vi "crio_RT_HX711.vi"() -> ()   [LabVIEW 2019]
uses:
  <vilib>/FPGAPlugInAG/cRIO-9074/niLvFpga_Open_cRIO-9074.vi
  <vilib>/rvi/interface/common/dynamic/niFpgaDynamicAddResources.vi
  <vilib>/Utility/error.llb/Error Cluster From Error Code.vi
  <vilib>/rvi/errors/niLvFpgaAdjustHostInterfaceError.vi
  <vilib>/FPGAPlugInAG/Dynamic/niLvFpga_Close_Dynamic.vi
  <vilib>/rvi/interface/nirviOpenFPGA/nirviOpenFPGA.xnode
  FPGA Bitfiles/gpass2_FPGATarget2_qweer_silS8sheR8k.lvbitx
  hx711/HX711.vi
  <vilib>/rvi/interface/nirviReadWriteControl/nirviReadWriteControl.xnode
  <vilib>/rvi/interface/nirviCloseFPGA/nirviCloseFPGA.xnode
  <vilib>/rvi/interface/Simulation/niFpgaSimulationCallBeginRW.vi
  NiFpgaLv.dll
  <vilib>/ptbypt/NI_PtbyPt.lvlib
panel:
  out "Offsetted Data":dbl(graph)
  out "Offsetted Data":dbl
  in  "Offset Bias":bool
  out "Computed Bias":dbl(graph)
  in  "Number of Samples for Offset Computation":i32=100
  out "Computed Bias":dbl format="%0.2f"
  out "Raw Data":i32(graph)
  in  "Gain/ChannelSelect":T1(ring)=enum."Channel A/Gain 64"
  out "HX711 Raw Data":i32
  in  "stop":bool
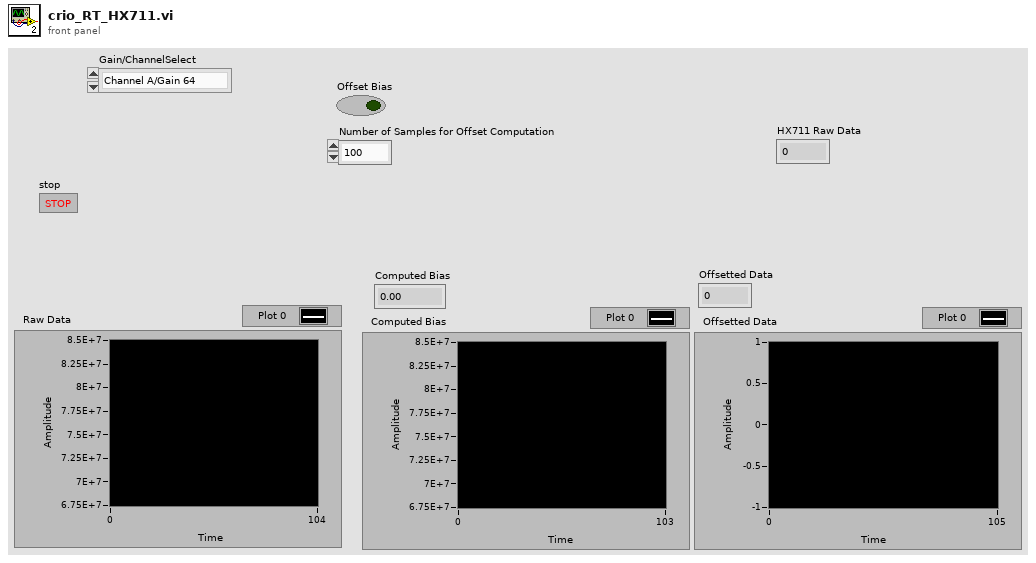
[diagram p1: front panel]
types:
  T1 = enum16{"Channel A/Gain 128", "Channel A/Gain 64", "Channel B/Gain 32"}
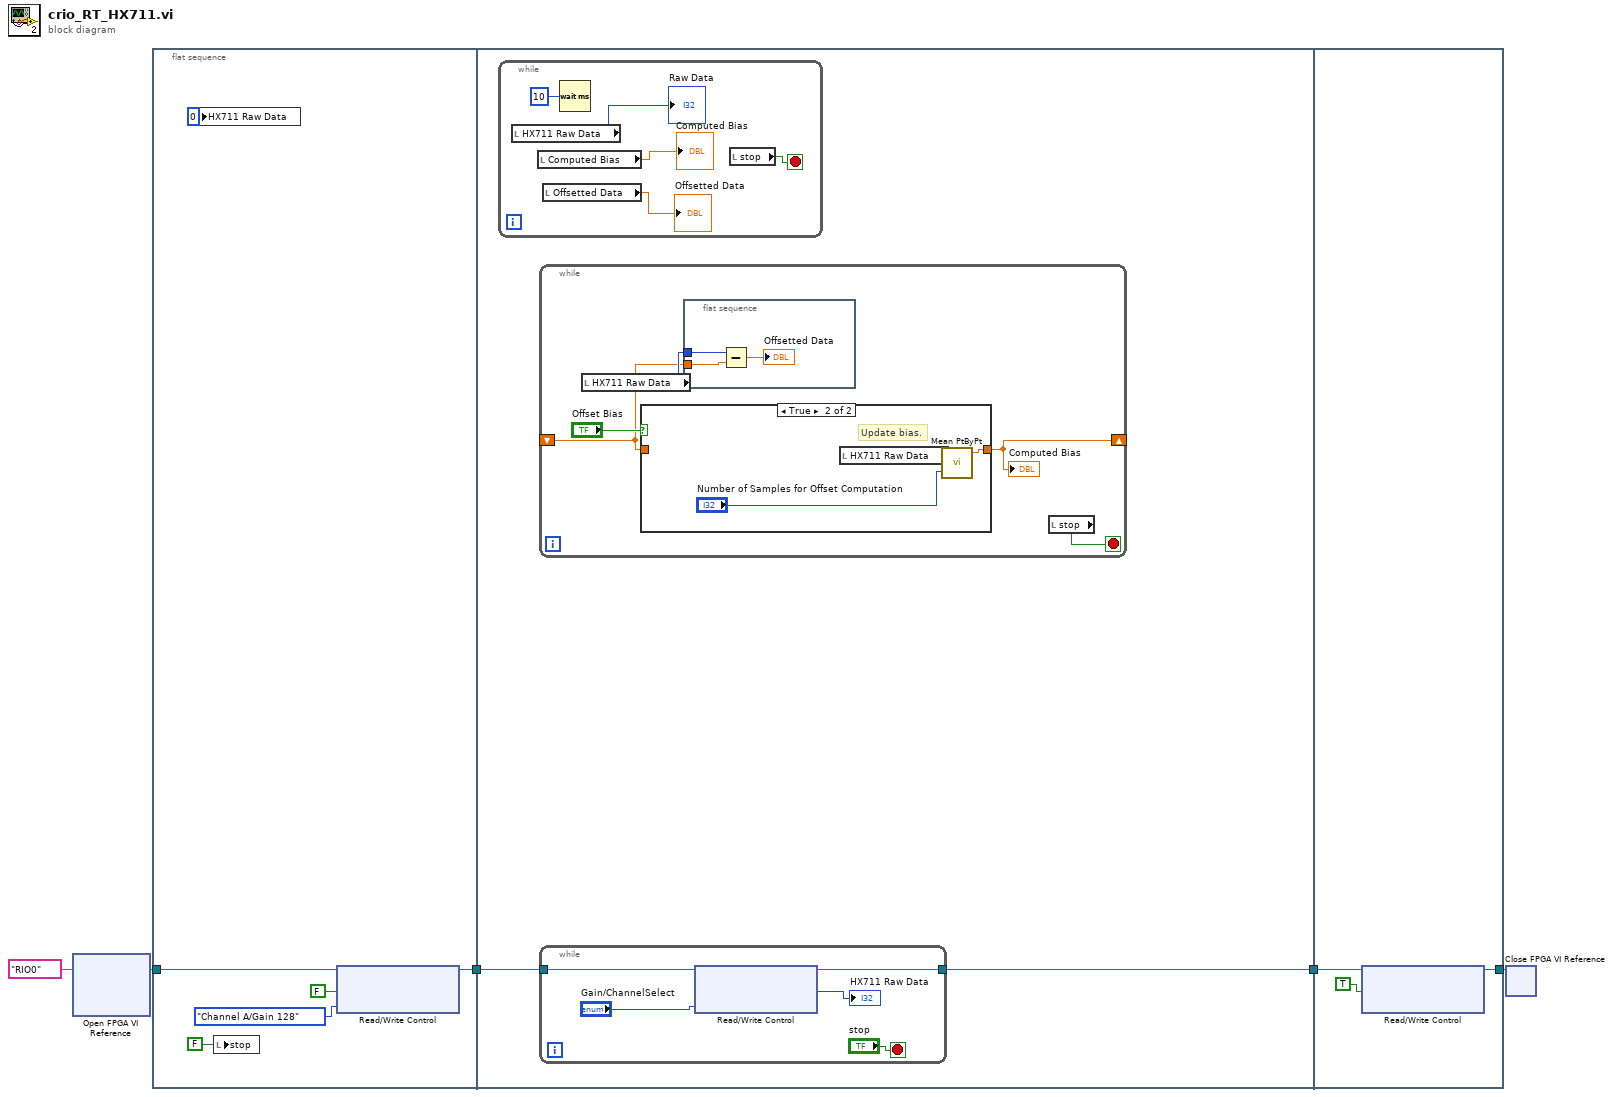
[diagram p0: block diagram]
diagram:
  n1 = xnode "Open FPGA VI Reference"("resource name"=tag "RIO0") -> ("FPGA VI Reference Out"=w4:refnum<k20>)  [unwired: 1 in, 1 out]
  n2 = flat-sequence {
    tunnel: w4 -> [w11]
    tunnel: [w9] -> w3
    tunnel: w3 -> [w12]
    tunnel: [w13] -> w2
    tunnel: w2 -> [w37]
    tunnel: [w36] -> w1
    frame #0 {
      n3 = local write "HX711 Raw Data"(0 ("Data")) -> ()
      n4 = local write "stop"(FALSE ("stop")) -> ()
      n5 = xnode "Read/Write Control"("FPGA VI Reference In"=w11, "stop"=FALSE, "Gain/ChannelSelect"=T1."Channel A/Gain 128") -> ("FPGA VI Reference Out"=w9:refnum<k20>)  [unwired: 1 in, 1 out]
    }
    frame #1 {
      n6 = while {
        stop <- w30 stop-if-true
        n7 = local read "HX711 Raw Data"() -> (→"Raw Data":i32)
        n8 = local read "Computed Bias"() -> (→"Computed Bias":dbl)
        n9 = local read "Offsetted Data"() -> (→"Offsetted Data":dbl)
        n10 = Wait (ms)(milliseconds to wait=u32 10) -> ()  [unwired: 1 out]
        n11 = local read "stop"() -> (w30:bool)
      }
      n12 = while {
        shift-right: [w16] -> _
        shift-left: _ -> [w14]
        stop <- w18 stop-if-true
        n13 = local read "HX711 Raw Data"() -> (w15:i32)
        n14 = case shown="True" "Offset Bias" {
          tunnel: [w22 w24] -> w16
          tunnel: w14 -> [w22 _]
          frame False {
            # "Stick with latest bias."
          }
          frame True {
            # "Update bias."
            n15 = local read "HX711 Raw Data"() -> (w25:i32)
            n16 = call <vilib>:"Mean PtByPt.vi"("x"=w25, "sample length"="Number of Samples for Offset Computation") -> ("mean"=w24:dbl)  [unwired: 2 in, 1 out]
          }
        }
        "Computed Bias" <- w16
        n17 = flat-sequence {
          tunnel: w15 -> [w21]
          tunnel: w14 -> [w20]
          frame #0 {
            n18 = Subtract(x=w21, y=w20) -> (x-y=→"Offsetted Data":dbl)
          }
        }
        n19 = local read "stop"() -> (w18:bool)
      }
      n20 = while {
        tunnel: w12 -> [w35]
        tunnel: [w32] -> w13
        stop <- "stop" stop-if-true
        n21 = xnode "Read/Write Control"("FPGA VI Reference In"=w35, "Gain/ChannelSelect"="Gain/ChannelSelect") -> ("FPGA VI Reference Out"=w32:refnum<k20>, "Data"=→"HX711 Raw Data":i32)  [unwired: 1 in, 1 out]
      }
    }
    frame #2 {
      n22 = xnode "Read/Write Control"("FPGA VI Reference In"=w37, "stop"=TRUE) -> ("FPGA VI Reference Out"=w36:refnum<k20>)  [unwired: 2 in, 1 out]
    }
  }
  n23 = xnode "Close FPGA VI Reference"("FPGA VI Reference In"=w1) -> ()  [unwired: 1 in, 1 out]
